vi "AnalyzeVIs.vi"(8 "error in (no error)":errorcluster) -> (0 "error out":errorcluster)   [LabVIEW 2020, in "CICD.lvlib"]
doc: "Run VI Analyzer."
uses:
  CICD.lvlib
  <vilib>/Wiresmith Technology/G CLI/CLI Class/CLI.lvclass
  <vilib>/Wiresmith Technology/G CLI/Argument Parser/Option Set Class/Option Set.lvclass
  <vilib>/Wiresmith Technology/G CLI/Argument Parser/Option Class/Argument Type.ctl
  <vilib>/Wiresmith Technology/G CLI/Argument Parser/Option Class/Option.lvclass
  <vilib>/Wiresmith Technology/G CLI/Argument Parser/Option Class/Option Configuration.ctl
  Private/Scope--enum.ctl
panel:
  out "-Scope":T1
  out "Output -ReportPath":path
  out "VIAnalyzer -ConfigPath":path
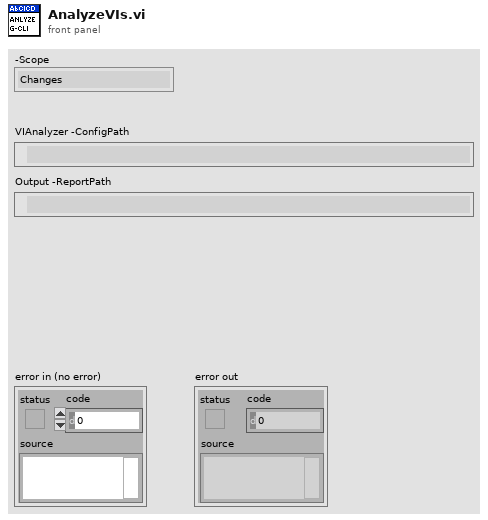
[diagram p1: front panel]
types:
  T1 = typedef "CICD.lvlib/Scope--enum.ctl" = enum16{"Changes", "All", "Folder"}
  T2 = typedef "Option Parser.lvlib/Option.lvclass/Option Configuration.ctl" = cluster{"Option Type":T3, "Option Labels":string[], "Key":string, "Description":string, "Required":bool, "Default Value":string}
  T3 = typedef "Option Parser.lvlib/Option.lvclass/Argument Type.ctl" = enum16{"flag", "value"}
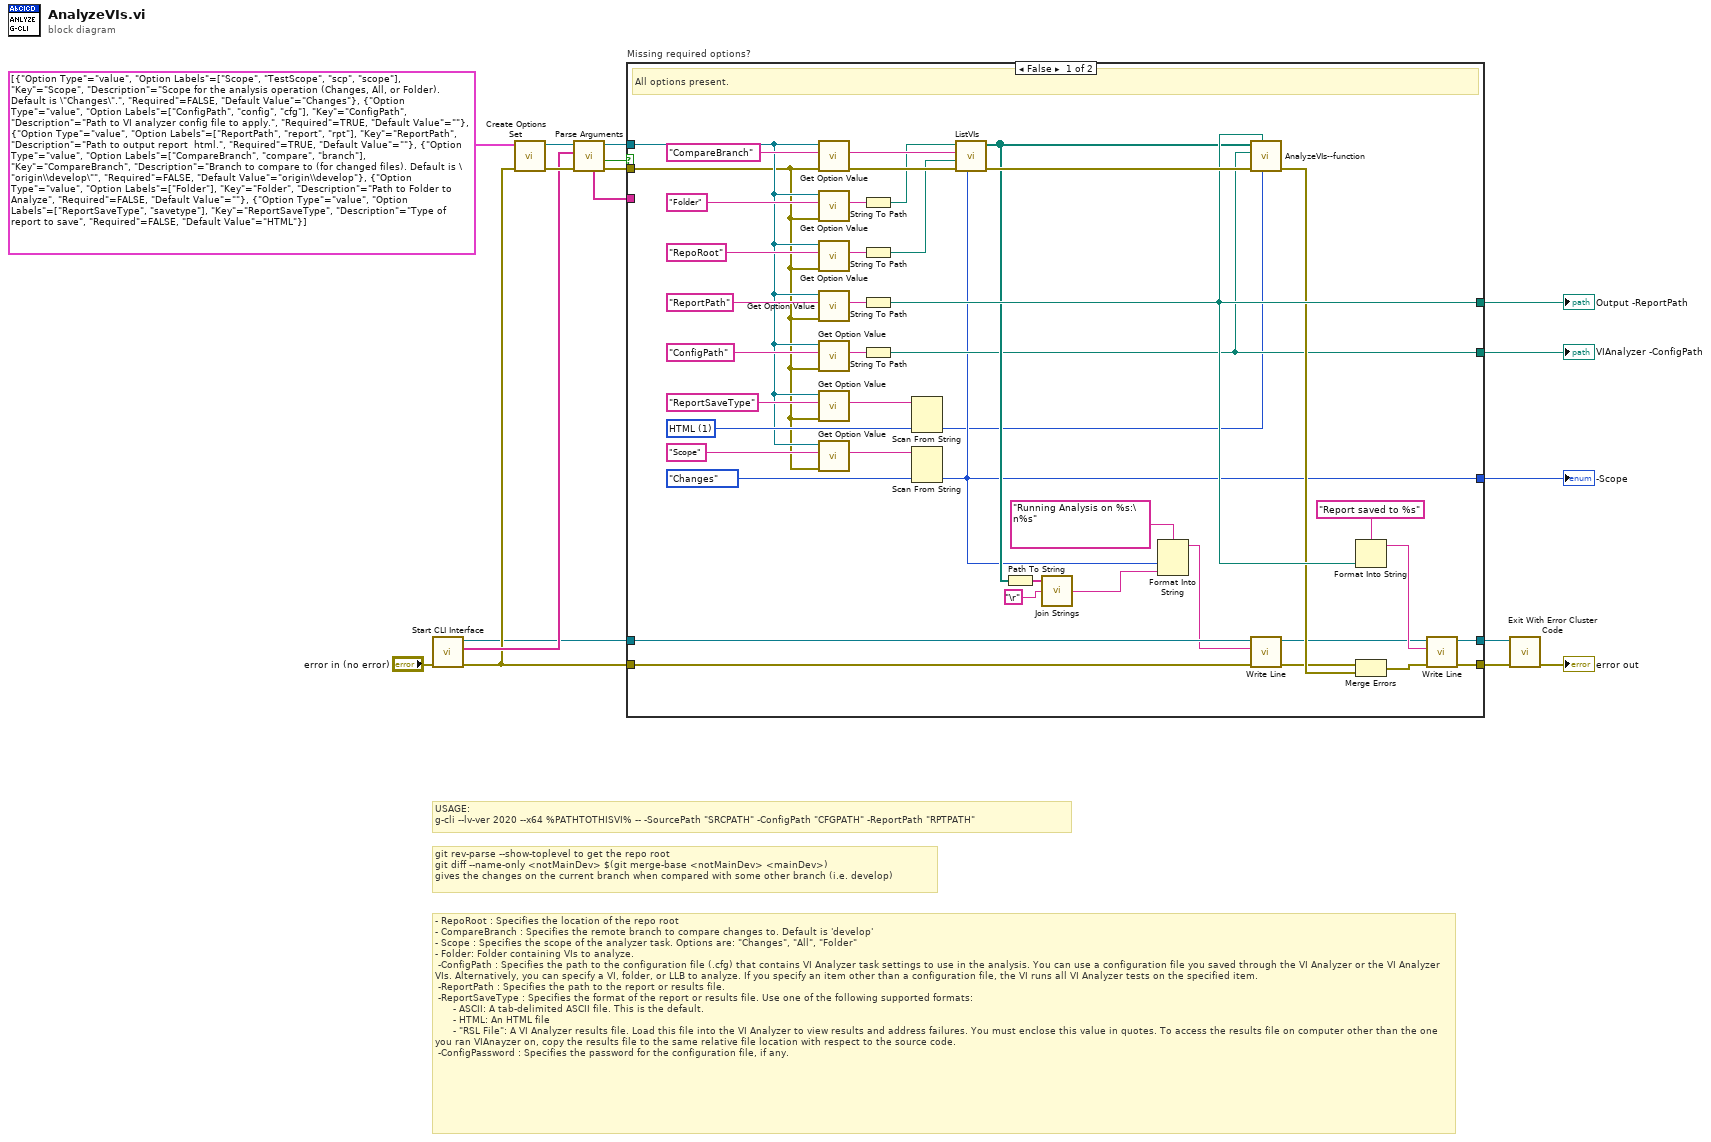
[diagram p0: block diagram]
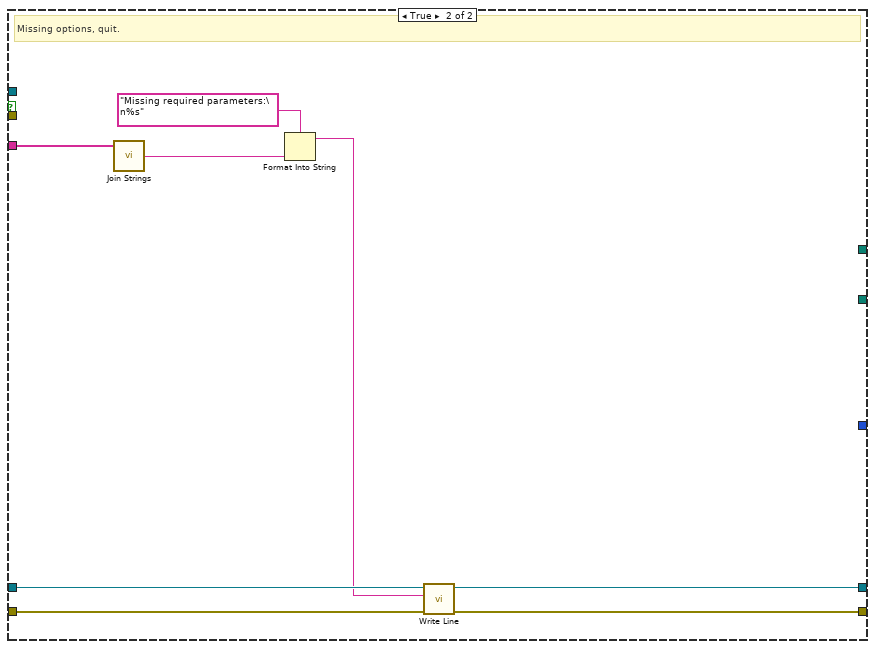
[diagram p2: hidden frame]
diagram:
  # "- RepoRoot : Specifies the location of the repo root\n- CompareBranch : Specifies the remote branch to compare changes to. Default is 'develop'\n- Scope : Specifies the scope of the analyzer task. Options are: \"Changes\", \"All\", \"Folder\"\n- Folder: Folder containing VIs to analyze.\n -ConfigPath : Specifies the path to the configuration file (.cfg) that contains VI Analyzer task settings to use in the analysis. You can use a configuration file you saved through the VI Analyzer or the VI Analyzer VIs. Alternatively, you can specify a VI, folder, or LLB to analyze. If you specify an item other than a configuration file, the VI runs all VI Analyzer tests on the specified item.\n -ReportPath : Specifies the path to the report or results file. \n -ReportSaveType : Specifies the format of the report or results file. Use one of the following supported formats:\n      - ASCII: A tab-delimited ASCII file. This is the default.\n      - HTML: An HTML file\n      - \"RSL File\": A VI Analyzer results file. Load this file into the VI Analyzer to view results and address failures. You must enclose this value in quotes. To access the results file on computer other than the one you ran VIAnayzer on, copy the results file to the same relative file location with respect to the source code.\n -ConfigPassword : Specifies the password for the configuration file, if any."
  # "git rev-parse --show-toplevel to get the repo root\ngit diff --name-only <notMainDev> $(git merge-base <notMainDev> <mainDev>)\ngives the changes on the current branch when compared with some other branch (i.e. develop)"
  # "USAGE:\ng-cli --lv-ver 2020 --x64 %PATHTOTHISVI% -- -SourcePath \"SRCPATH\" -ConfigPath \"CFGPATH\" -ReportPath \"RPTPATH\""
  n1 = call <vilib>:"Start CLI Interface.vi"("error in (no error)"="error in (no error)") -> ("error out"=w7:errorcluster, "Custom Parameters"=w12:string[], "CLI out"=w6:refnum<class "CLI.lvclass">)  [unwired: 7 in, 1 out]
  n2 = call <vilib>:"Create Options Set.vi"("error in (no error)"=w7, "Options"=T2[] [{"Option Type"=enum."value", "Option Labels"=["Scope", "TestScope", "scp", "scope"], "Key"="Scope", "Description"="Scope for the analysis operation (Changes, All, or Folder). Default is \"Changes\".", "Required"=FALSE, "Default Value"="Changes"}, {"Option Type"=enum."value", "Option Labels"=["ConfigPath", "config", "cfg"], "Key"="ConfigPath", "Description"="Path to VI analyzer config file to apply.", "Required"=TRUE, "Default Value"=""}, {"Option Type"=enum."value", "Option Labels"=["ReportPath", "report", "rpt"], "Key"="ReportPath", "Description"="Path to output report  html.", "Required"=TRUE, "Default Value"=""}, {"Option Type"=enum."value", "Option Labels"=["CompareBranch", "compare", "branch"], "Key"="CompareBranch", "Description"="Branch to compare to (for changed files). Default is \"origin\\develop\"", "Required"=FALSE, "Default Value"="origin\\develop"}, {"Option Type"=enum."value", "Option Labels"=["Folder"], "Key"="Folder", "Description"="Path to Folder to Analyze", "Required"=FALSE, "Default Value"=""}, {"Option Type"=enum."value", "Option Labels"=["ReportSaveType", "savetype"], "Key"="ReportSaveType", "Description"="Type of report to save", "Required"=FALSE, "Default Value"="HTML"}]) -> ("error out"=w13:errorcluster, "Option Set out"=w14:refnum<class "Option Set.lvclass">)  [unwired: 8 in]
  n3 = call <vilib>:"Parse Arguments.vi"("error in (no error)"=w13, "Arguments"=w12, "Option Set in"=w14) -> ("error out"=w10:errorcluster, "Missing Options"=w8:bool, "Option Set out"=w11:refnum<class "Option Set.lvclass">, "Missing Option Keys"=w3:string[])  [unwired: 5 in]
  n4 = case "Missing required options?" shown="False" w8 {
    tunnel: [w51 w66] -> w16
    tunnel: w11 -> [w19 _]
    tunnel: w10 -> [w18 _]
    tunnel: w7 -> [w53 w67]
    tunnel: w6 -> [w50 w65]
    tunnel: [w47 _] -> w5
    tunnel: [w30 _] -> w4
    tunnel: w3 -> [_ w63]
    tunnel: [w46 w60] -> w2
    tunnel: [w24 _] -> w1
    frame False {
      w22 = u16 1 items=["ASCII", "HTML", "RSL File"] ("Report Save Type (ASCII)")
      # "All options present."
      n5 = call <vilib>:"Get Option Value.vi"("error in (no error)"=w18, "Option Key"="CompareBranch", "Option Set in"=w19) -> ("error out"=w42:errorcluster, "Value"=w35:string)  [unwired: 5 in, 2 out]
      n6 = call <vilib>:"Get Option Value.vi"("error in (no error)"=w18, "Option Key"="Folder", "Option Set in"=w19) -> ("Value"=w57:string)  [unwired: 5 in, 3 out]
      n7 = call <vilib>:"Get Option Value.vi"("error in (no error)"=w18, "Option Key"="RepoRoot", "Option Set in"=w19) -> ("Value"=w27:string)  [unwired: 5 in, 3 out]
      n8 = call <vilib>:"Get Option Value.vi"("error in (no error)"=w18, "Option Key"="ReportPath", "Option Set in"=w19) -> ("Value"=w56:string)  [unwired: 5 in, 3 out]
      n9 = call <vilib>:"Get Option Value.vi"("error in (no error)"=w18, "Option Key"="ConfigPath", "Option Set in"=w19) -> ("Value"=w31:string)  [unwired: 5 in, 3 out]
      n10 = call <vilib>:"Get Option Value.vi"("error in (no error)"=w18, "Option Key"="ReportSaveType", "Option Set in"=w19) -> ("Value"=w21:string)  [unwired: 5 in, 3 out]
      n11 = call <vilib>:"Get Option Value.vi"("error in (no error)"=w18, "Option Key"="Scope", "Option Set in"=w19) -> ("Value"=w29:string)  [unwired: 5 in, 3 out]
      n12 = String To Path(string=w57) -> (path=w32:path)
      n13 = String To Path(string=w27) -> (path=w26:path)
      n14 = String To Path(string=w56) -> (path=w47:path)
      n15 = String To Path(string=w31) -> (path=w30:path)
      n16 = Scan From String(input string=w21, default 1=w22) -> (output 1=w20:u16)  [unwired: 3 in, 3 out]
      n17 = Scan From String(input string=w29, default 1=Scope--enum."Changes" ("-TestScope")) -> (output 1=w24:T1)  [unwired: 3 in, 3 out]
      n18 = call "ListVIs.vi"("Scope"=w24, "error in"=w42, "RepoRoot"=w26, "Remote Branch to Compare"=w35, "Folder Path"=w32) -> ("error out"=w48:errorcluster, "VIs"=w39:path[])  [unwired: 5 in]
      n19 = Path To String(path=w39) -> (string=w38:string[])
      n20 = call <vilib>:"Join Strings.vi"("Separator (,)"="\r", "Strings In"=w38) -> ("String"=w34:string)  [unwired: 1 in]
      n21 = Format Into String(format string="Running Analysis on %s:\n%s", w24, w34) -> (resulting string=w25:string)  [unwired: 2 in, 1 out]
      n22 = call "AnalyzeVIs--function.vi"("Report Save Type (ASCII)"=w20, "ReportPath"=w47, "error in"=w48, "VIANConfig"=w30, "VIs to Analyze"=w39) -> ("error out"=w44:errorcluster)  [unwired: 5 in, 1 out]
      n23 = call <vilib>:"Write Line.vi"("error in (no error)"=w53, "Text to Write"=w25, "CLI in"=w50) -> ("error out"=w41:errorcluster, "CLI out"=w40:refnum<class "CLI.lvclass">)  [unwired: 7 in]
      n24 = Format Into String(format string="Report saved to %s", w47) -> (resulting string=w43:string)  [unwired: 2 in, 1 out]
      n25 = Merge Errors(w41, w44) -> (w45:errorcluster)
      n26 = call <vilib>:"Write Line.vi"("error in (no error)"=w45, "Text to Write"=w43, "CLI in"=w40) -> ("error out"=w51:errorcluster, "CLI out"=w46:refnum<class "CLI.lvclass">)  [unwired: 7 in]
    }
    frame True {
      # "Missing options, quit."
      n27 = call <vilib>:"Join Strings.vi"("Strings In"=w63) -> ("String"=w64:string)  [unwired: 2 in]
      n28 = Format Into String(format string="Missing required parameters:\n%s" ("Text to Write"), w64) -> (resulting string=w61:string)  [unwired: 2 in, 1 out]
      n29 = call <vilib>:"Write Line.vi"("error in (no error)"=w67, "Text to Write"=w61, "CLI in"=w65) -> ("error out"=w66:errorcluster, "CLI out"=w60:refnum<class "CLI.lvclass">)  [unwired: 7 in]
    }
  }
  "VIAnalyzer -ConfigPath" <- w4
  "Output -ReportPath" <- w5
  "-Scope" <- w1
  n30 = call <vilib>:"Exit With Error Cluster Code.vi"("error in (no error)"=w16, "CLI in"=w2) -> ("error out"=→"error out":errorcluster)  [unwired: 9 in]
